vi "stop_FGV.vi"(7 "comandos":enum16{"Iniciar", "Parar", "Parar?"}(ring)=enum."Parar?", 8 "error in (no error)":errorcluster) -> (0 "error out":errorcluster, 4 "parar?":bool)   [LabVIEW 2017]
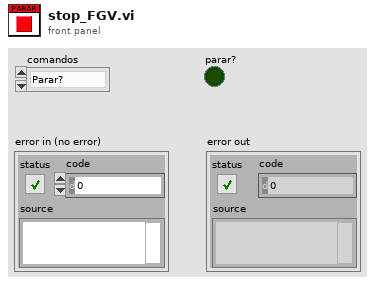
[diagram p1: front panel]
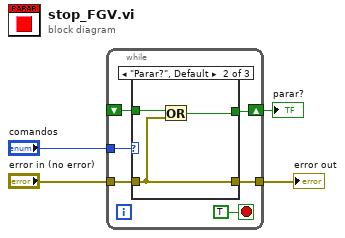
[diagram p0: block diagram]
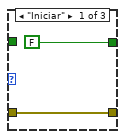
[diagram p2: hidden frame]
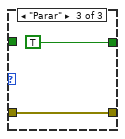
[diagram p3: hidden frame]
diagram:
  n1 = while {
    tunnel: "error in (no error)" -> [w6]
    tunnel: [w5] -> w3
    tunnel: "comandos" -> [w9]
    shift-right: [w8] -> w1
    shift-left: _ -> [w7]
    stop <- TRUE stop-if-true
    n2 = case shown="\"Parar?\", Default" w9 {
      tunnel: [FALSE w14 TRUE] -> w8
      tunnel: w7 -> [_ w15 _]
      tunnel: w6 -> [w11 w13 w16]
      tunnel: [w11 w13 w16] -> w5
      frame "Iniciar" {
      }
      frame "Parar?", Default {
        n3 = Or(x=w15, y=w13) -> (x .or. y?=w14:bool)
      }
      frame "Parar" {
      }
    }
  }
  "error out" <- w3
  "parar?" <- w1
